vi "Put-Ball-Pro_Api.vi"(8 "Error In":errorcluster, 10 "HiTechnicColorSensorV2 Ref In":cluster{"I2C Ref Out":T2}, 11 "輸出顏色-位置":T1(array[cluster])) -> (0 "Error Out":errorcluster, 3 "HiTechnicColorSensorV2 Ref Out":cluster{"I2C Ref Out":T2})   [LabVIEW 2019]
uses:
  <vilib>/myRIO/Instrument Drivers/Onboard IO/I2C/typedefs/I2C Reference.ctl
  <vilib>/myRIO/Common/Instrument Driver Framework/Utilities/typedefs/myRIO Generic Hardware Reference.ctl
  <vilib>/myRIO/Common/Instrument Driver Framework/Utilities/typedefs/Hardware Version Enum.ctl
  <vilib>/myRIO/Common/Instrument Driver Framework/Utilities/typedefs/myRIO v1.0 Reference.ctl
  <vilib>/myRIO/Common/Instrument Driver Framework/Utilities/typedefs/Generic FPGA Reference.ctl
  <vilib>/myRIO/Common/Instrument Driver Framework/myRIO v1.0/I2C/typedefs/I2C Channels Enum.ctl
  <vilib>/myRIO/Instrument Drivers/Onboard IO/I2C/typedefs/I2C Configuration.ctl
  <vilib>/myRIO/Instrument Drivers/Onboard IO/I2C/typedefs/I2C Transfer Rate.ctl
  Variable/Go-Home.vi
  <vilib>/myRIO/Instrument Drivers/Onboard IO/I2C/I2C.lvlib
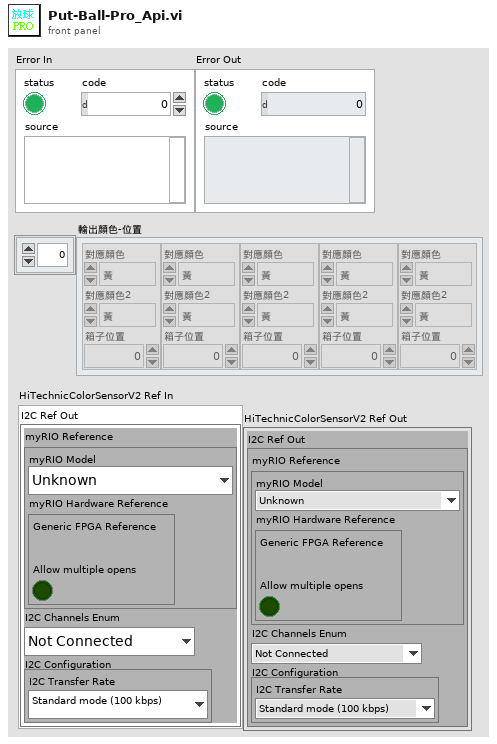
[diagram p1: front panel]
types:
  T1 = cluster{"對應顏色":enum16{"黃", "紅", "綠", "藍", "黑", "無"}, "對應顏色2":enum16{"黃", "紅", "綠", "藍", "黑", "無"}, "箱子位置":i32}[]
  T2 = typedef "I2C.lvlib/I2C Reference.ctl" = cluster{"myRIO Reference":T3, "I2C Channels Enum":T7, "I2C Configuration":T8}
  T3 = typedef "myRIO Generic Hardware Reference.ctl" = cluster{"myRIO Model":T4, "myRIO Hardware Reference":T5}
  T4 = typedef "Hardware Version Enum.ctl" = enum16{"Unknown", "myRIO-1900", "myRIO-1950", "roboRIO", "NI ELVIS RIO CM", "ELVIS III"}
  T5 = typedef "myRIO v1.0 Reference.ctl" = cluster{"Generic FPGA Reference":T6, "Allow multiple opens":bool}
  T6 = typedef "Generic FPGA Reference.ctl" = refnum<k20>
  T7 = typedef "I2C Channels Enum.ctl" = enum16{"Not Connected", "A/I2C", "B/I2C", "I2C/I2C"}
  T8 = typedef "I2C.lvlib/I2C Configuration.ctl" = cluster{"I2C Transfer Rate":T9}
  T9 = typedef "I2C.lvlib/I2C Transfer Rate.ctl" = enum16{"Standard mode (100 kbps)", "Fast mode (400 kbps)"}
  T10 = enum16{"前", "後", "オ", "右", "無", "0", "1", "2", "3", "4", "5", "6", "7"}
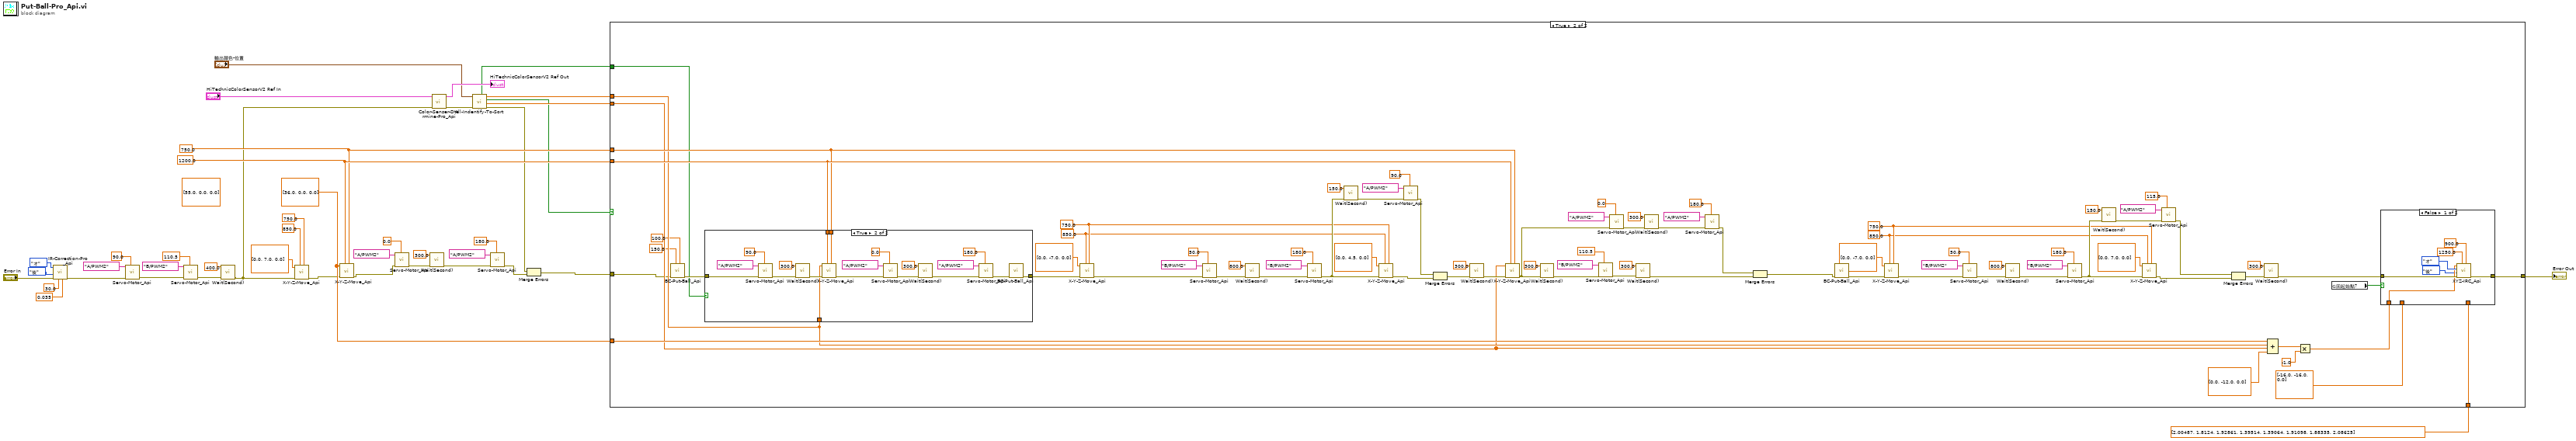
[diagram p0: block diagram]
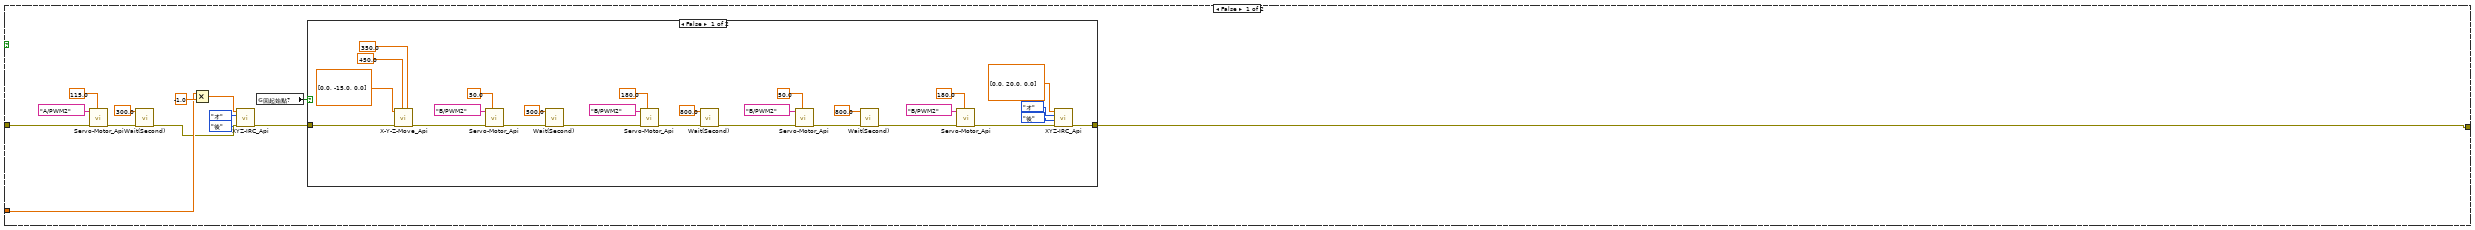
[diagram p2: hidden frame]
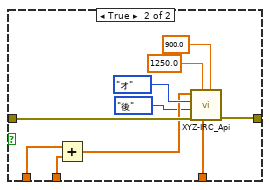
[diagram p5: hidden frame]
diagram:
  (unwired) dbl[] [55.0, 0.0, 0.0] ("X-Y-Z移動")
  w29 = 750.0 ("加速度")
  w30 = 1200.0 ("最高速")
  w32 = dbl[] [36.0, 0.0, 0.0] ("X-Y-Z移動")
  n1 = call "IR-Correction-Pro_Api.vi"("ExitRange"=0.035, "精準度"=30.0, "Error In"="Error In", "副邊校正"=T10."後", "主編校正"=enum16{"前", "後", "オ", "右", "無"}."オ") -> ("Error Out"=w2:errorcluster)  [unwired: 6 in]
  n2 = call "Servo-Motor_Api.vi"("角度"=90.0, "Error In"=w2, "伺服馬達角位"=tag "A/PWM2") -> ("Error Out"=w3:errorcluster)  [unwired: 8 in]
  n3 = call "Servo-Motor_Api.vi"("角度"=110.5, "Error In"=w3, "伺服馬達角位"=tag "B/PWM2") -> ("Error Out"=w10:errorcluster)  [unwired: 8 in]
  n4 = call "Wait(Second).vi"("Error In"=w10, "等待秒數(3000毫秒)"=400.0) -> ("Error Out"=w9:errorcluster)  [unwired: 9 in]
  n5 = call "X-Y-Z-Move_Api.vi"("加速度"=750.0, "最高速"=850.0, "Error In"=w9, "X-Y-Z移動"=dbl[] [0.0, 7.0, 0.0]) -> ("Error Out"=w22:errorcluster)  [unwired: 6 in, 1 out]
  n6 = call "X-Y-Z-Move_Api.vi"("加速度"=w29, "最高速"=w30, "Error In"=w22, "X-Y-Z移動"=w32) -> ("Error Out"=w6:errorcluster)  [unwired: 6 in, 1 out]
  n7 = call "Servo-Motor_Api.vi"("角度"=0.0, "Error In"=w6, "伺服馬達角位"=tag "A/PWM2") -> ("Error Out"=w37:errorcluster)  [unwired: 8 in]
  n8 = call "Wait(Second).vi"("Error In"=w37, "等待秒數(3000毫秒)"=300.0) -> ("Error Out"=w33:errorcluster)  [unwired: 9 in]
  n9 = call "Color-Senser-Dtermine-Pro_Api.vi"("Error In"=w9, "HiTechnicColorSensorV2 Ref In"="HiTechnicColorSensorV2 Ref In") -> ("Error Out"=w21:errorcluster, "HiTechnicColorSensorV2 Ref Out"=→"HiTechnicColorSensorV2 Ref Out":cluster{"I2C Ref Out":T2})  [unwired: 4 in, 4 out]
  n10 = call "All-Indentify-To-Sort.vi"("Error In"=w21, "輸出顏色-位置"="輸出顏色-位置") -> ("Error Out"=w20:errorcluster, "輸出移動值2"=w16:dbl[], "執行放球?"=w15:bool, "輸出移動值"=w17:dbl[], "執行補值、校正?"=w18:bool)  [unwired: 5 in]
  n11 = call "Servo-Motor_Api.vi"("角度"=180.0, "Error In"=w33, "伺服馬達角位"=tag "A/PWM2") -> ("Error Out"=w25:errorcluster)  [unwired: 8 in]
  n12 = Merge Errors(w20, w25) -> (w31:errorcluster)
  n13 = case shown="True" w15 {
    tunnel: [w46 w136] -> w8
    tunnel: w32 -> [w54 w131]
    tunnel: w31 -> [w45 w105]
    tunnel: w30 -> [_ w118]
    tunnel: w29 -> [_ w117]
    tunnel: w18 -> [_ w111]
    tunnel: w17 -> [_ w110]
    tunnel: w16 -> [_ w109]
    tunnel: dbl[] [2.00487, 1.8124, 1.92861, 1.39514, 1.39064, 1.91098, 1.88335, 2.08625] ("目標電壓") -> [_ w85]
    frame False {
      n14 = call "Servo-Motor_Api.vi"("角度"=115.0, "Error In"=w45, "伺服馬達角位"=tag "A/PWM2") -> ("Error Out"=w48:errorcluster)  [unwired: 8 in]
      n15 = call "Wait(Second).vi"("Error In"=w48, "等待秒數(3000毫秒)"=300.0) -> ("Error Out"=w47:errorcluster)  [unwired: 9 in]
      n16 = Multiply(x=w54, y=-1.0) -> (x*y=w56:dbl[])
      n17 = call "XYZ-IRC_Api.vi"("Error"=w47, "副邊校正"=T10."後", "主編校正"=enum16{"前", "後", "オ", "右", "無"}."オ", "X-Y-Z移動"=w56) -> ("Error Out"=w52:errorcluster)  [unwired: 7 in]
      n18 = global read "Go-Home.vi" "回起始點?"() -> (w44:bool)
      n19 = case shown="False" w44 {
        tunnel: w52 -> [w67 w84]
        tunnel: [w64 w84] -> w46
        frame False {
          n20 = call "X-Y-Z-Move_Api.vi"("加速度"=350.0, "最高速"=450.0, "Error In"=w67, "X-Y-Z移動"=dbl[] [0.0, -15.0, 0.0]) -> ("Error Out"=w68:errorcluster)  [unwired: 6 in, 1 out]
          n21 = call "Servo-Motor_Api.vi"("角度"=50.0, "Error In"=w68, "伺服馬達角位"=tag "B/PWM2") -> ("Error Out"=w80:errorcluster)  [unwired: 8 in]
          n22 = call "Wait(Second).vi"("Error In"=w80, "等待秒數(3000毫秒)"=500.0) -> ("Error Out"=w75:errorcluster)  [unwired: 9 in]
          n23 = call "Servo-Motor_Api.vi"("角度"=180.0, "Error In"=w75, "伺服馬達角位"=tag "B/PWM2") -> ("Error Out"=w74:errorcluster)  [unwired: 8 in]
          n24 = call "Wait(Second).vi"("Error In"=w74, "等待秒數(3000毫秒)"=800.0) -> ("Error Out"=w69:errorcluster)  [unwired: 9 in]
          n25 = call "Servo-Motor_Api.vi"("角度"=50.0, "Error In"=w69, "伺服馬達角位"=tag "B/PWM2") -> ("Error Out"=w73:errorcluster)  [unwired: 8 in]
          n26 = call "Wait(Second).vi"("Error In"=w73, "等待秒數(3000毫秒)"=800.0) -> ("Error Out"=w61:errorcluster)  [unwired: 9 in]
          n27 = call "Servo-Motor_Api.vi"("角度"=180.0, "Error In"=w61, "伺服馬達角位"=tag "B/PWM2") -> ("Error Out"=w60:errorcluster)  [unwired: 8 in]
          n28 = call "XYZ-IRC_Api.vi"("Error"=w60, "副邊校正"=T10."後", "主編校正"=enum16{"前", "後", "オ", "右", "無"}."オ", "X-Y-Z移動"=dbl[] [0.0, 20.0, 0.0]) -> ("Error Out"=w64:errorcluster)  [unwired: 7 in]
        }
        frame True {
        }
      }
    }
    frame True {
      w115 = 750.0 ("加速度")
      w114 = 850.0 ("最高速")
      w113 = 750.0 ("加速度")
      w112 = 850.0 ("最高速")
      n29 = call "BC-Put-Ball_Api.vi"("加速度"=100.0, "最高速"=150.0, "Error In"=w105) -> ("Error Out"=w165:errorcluster)  [unwired: 8 in]
      n30 = case shown="True" w111 {
        tunnel: w165 -> [w166 w183]
        tunnel: [w166 w170] -> w151
        tunnel: w110 -> [_ w179]
        tunnel: w118 -> [_ w168]
        tunnel: w117 -> [_ w167]
        frame False {
        }
        frame True {
          n31 = call "Servo-Motor_Api.vi"("角度"=90.0, "Error In"=w183, "伺服馬達角位"=tag "A/PWM2") -> ("Error Out"=w181:errorcluster)  [unwired: 8 in]
          n32 = call "Wait(Second).vi"("Error In"=w181, "等待秒數(3000毫秒)"=300.0) -> ("Error Out"=w180:errorcluster)  [unwired: 9 in]
          n33 = call "X-Y-Z-Move_Api.vi"("加速度"=w167, "最高速"=w168, "Error In"=w180, "X-Y-Z移動"=w179) -> ("Error Out"=w169:errorcluster)  [unwired: 6 in, 1 out]
          n34 = call "Servo-Motor_Api.vi"("角度"=0.0, "Error In"=w169, "伺服馬達角位"=tag "A/PWM2") -> ("Error Out"=w173:errorcluster)  [unwired: 8 in]
          n35 = call "Wait(Second).vi"("Error In"=w173, "等待秒數(3000毫秒)"=300.0) -> ("Error Out"=w178:errorcluster)  [unwired: 9 in]
          n36 = call "Servo-Motor_Api.vi"("角度"=180.0, "Error In"=w178, "伺服馬達角位"=tag "A/PWM2") -> ("Error Out"=w177:errorcluster)  [unwired: 8 in]
          n37 = call "BC-Put-Ball_Api.vi"("Error In"=w177) -> ("Error Out"=w170:errorcluster)  [unwired: 10 in]
        }
      }
      n38 = call "X-Y-Z-Move_Api.vi"("加速度"=w113, "最高速"=w112, "Error In"=w151, "X-Y-Z移動"=dbl[] [0.0, -7.0, 0.0]) -> ("Error Out"=w108:errorcluster)  [unwired: 6 in, 1 out]
      n39 = call "Servo-Motor_Api.vi"("角度"=50.0, "Error In"=w108, "伺服馬達角位"=tag "B/PWM2") -> ("Error Out"=w156:errorcluster)  [unwired: 8 in]
      n40 = call "Wait(Second).vi"("Error In"=w156, "等待秒數(3000毫秒)"=800.0) -> ("Error Out"=w153:errorcluster)  [unwired: 9 in]
      n41 = call "Servo-Motor_Api.vi"("角度"=180.0, "Error In"=w153, "伺服馬達角位"=tag "B/PWM2") -> ("Error Out"=w122:errorcluster)  [unwired: 8 in]
      n42 = call "Wait(Second).vi"("Error In"=w122, "等待秒數(3000毫秒)"=150.0) -> ("Error Out"=w160:errorcluster)  [unwired: 9 in]
      n43 = call "X-Y-Z-Move_Api.vi"("加速度"=w113, "最高速"=w112, "Error In"=w122, "X-Y-Z移動"=dbl[] [0.0, 4.5, 0.0]) -> ("Error Out"=w119:errorcluster)  [unwired: 6 in, 1 out]
      n44 = call "Servo-Motor_Api.vi"("角度"=90.0, "Error In"=w160, "伺服馬達角位"=tag "A/PWM2") -> ("Error Out"=w120:errorcluster)  [unwired: 8 in]
      n45 = Merge Errors(w120, w119) -> (w121:errorcluster)
      n46 = call "Wait(Second).vi"("Error In"=w121, "等待秒數(3000毫秒)"=300.0) -> ("Error Out"=w129:errorcluster)  [unwired: 9 in]
      n47 = call "X-Y-Z-Move_Api.vi"("加速度"=w117, "最高速"=w118, "Error In"=w129, "X-Y-Z移動"=w109) -> ("Error Out"=w86:errorcluster)  [unwired: 6 in, 1 out]
      n48 = call "Wait(Second).vi"("Error In"=w86, "等待秒數(3000毫秒)"=300.0) -> ("Error Out"=w98:errorcluster)  [unwired: 9 in]
      n49 = call "Servo-Motor_Api.vi"("角度"=110.5, "Error In"=w98, "伺服馬達角位"=tag "B/PWM2") -> ("Error Out"=w97:errorcluster)  [unwired: 8 in]
      n50 = call "Servo-Motor_Api.vi"("角度"=0.0, "Error In"=w86, "伺服馬達角位"=tag "A/PWM2") -> ("Error Out"=w92:errorcluster)  [unwired: 8 in]
      n51 = call "Wait(Second).vi"("Error In"=w97, "等待秒數(3000毫秒)"=300.0) -> ("Error Out"=w96:errorcluster)  [unwired: 9 in]
      n52 = call "Wait(Second).vi"("Error In"=w92, "等待秒數(3000毫秒)"=300.0) -> ("Error Out"=w88:errorcluster)  [unwired: 9 in]
      n53 = call "Servo-Motor_Api.vi"("角度"=180.0, "Error In"=w88, "伺服馬達角位"=tag "A/PWM2") -> ("Error Out"=w87:errorcluster)  [unwired: 8 in]
      n54 = Merge Errors(w87, w96) -> (w95:errorcluster)
      n55 = call "BC-Put-Ball_Api.vi"("Error In"=w95) -> ("Error Out"=w137:errorcluster)  [unwired: 10 in]
      n56 = call "X-Y-Z-Move_Api.vi"("加速度"=w115, "最高速"=w114, "Error In"=w137, "X-Y-Z移動"=dbl[] [0.0, -7.0, 0.0]) -> ("Error Out"=w107:errorcluster)  [unwired: 6 in, 1 out]
      n57 = call "Servo-Motor_Api.vi"("角度"=50.0, "Error In"=w107, "伺服馬達角位"=tag "B/PWM2") -> ("Error Out"=w146:errorcluster)  [unwired: 8 in]
      n58 = call "Wait(Second).vi"("Error In"=w146, "等待秒數(3000毫秒)"=800.0) -> ("Error Out"=w149:errorcluster)  [unwired: 9 in]
      n59 = call "Servo-Motor_Api.vi"("角度"=180.0, "Error In"=w149, "伺服馬達角位"=tag "B/PWM2") -> ("Error Out"=w123:errorcluster)  [unwired: 8 in]
      n60 = call "Wait(Second).vi"("Error In"=w123, "等待秒數(3000毫秒)"=150.0) -> ("Error Out"=w142:errorcluster)  [unwired: 9 in]
      n61 = call "X-Y-Z-Move_Api.vi"("加速度"=w115, "最高速"=w114, "Error In"=w123, "X-Y-Z移動"=dbl[] [0.0, 7.0, 0.0]) -> ("Error Out"=w124:errorcluster)  [unwired: 6 in, 1 out]
      n62 = call "Servo-Motor_Api.vi"("角度"=115.0, "Error In"=w142, "伺服馬達角位"=tag "A/PWM2") -> ("Error Out"=w125:errorcluster)  [unwired: 8 in]
      n63 = Merge Errors(w125, w124) -> (w126:errorcluster)
      n64 = call "Wait(Second).vi"("Error In"=w126, "等待秒數(3000毫秒)"=300.0) -> ("Error Out"=w127:errorcluster)  [unwired: 9 in]
      n65 = Compound Arithmetic op=ADD(w131, w110, w109, dbl[] [0.0, -12.0, 0.0] ("value")) -> (w135:dbl[])
      n66 = Multiply(x=w135, y=-1.0) -> (x*y=w134:dbl[])
      n67 = global read "Go-Home.vi" "回起始點?"() -> (w106:bool)
      n68 = case shown="False" w106 {
        tunnel: w127 -> [w191 w199]
        tunnel: [w190 w198] -> w136
        tunnel: w134 -> [w189 w202]
        tunnel: dbl[] [-16.0, -16.0, 0.0] ("X-Y-Z移動") -> [_ w201]
        tunnel: w85 -> [_ w195]
        frame False {
          n69 = call "XYZ-IRC_Api.vi"("加速度"=900.0, "最高速"=1250.0, "Error"=w191, "副邊校正"=T10."後", "主編校正"=enum16{"前", "後", "オ", "右", "無"}."オ", "X-Y-Z移動"=w189) -> ("Error Out"=w190:errorcluster)  [unwired: 5 in]
        }
        frame True {
          n70 = Add(x=w202, y=w201) -> (x+y=w197:dbl[])
          n71 = call "XYZ-IRC_Api.vi"("加速度"=900.0, "目標電壓"=w195, "最高速"=1250.0, "Error"=w199, "副邊校正"=T10."後", "主編校正"=enum16{"前", "後", "オ", "右", "無"}."オ", "X-Y-Z移動"=w197) -> ("Error Out"=w198:errorcluster)  [unwired: 4 in]
        }
      }
    }
  }
  "Error Out" <- w8
